vi "Get Exclusions.vi"(8 "error in (no error)":errorcluster, 11 "NI_AB_API_Build in":refnum<class "NI_AB_API_Build.lvclass">) -> (0 "error out":errorcluster, 1 "Disconnect inline subVIs":bool, 2 "Exclusions":T1, 3 "NI_AB_API_Build out":refnum<class "NI_AB_API_Build.lvclass">, 4 "Exclude dependent shared libraries":bool, 6 "Exclude dependent packed libraries":bool)   [LabVIEW 2020, in "NI_AB_API_Build.lvclass"]
uses:
  <vilib>/AppBuilder/AB_API/Build/NI_AB_API_Build.lvclass
  <vilib>/AppBuilder/AB_API/common/AB_API Primary Exclusions.ctl
  <vilib>/AppBuilder/AB_API/Build/NI_AB_API_Build.lvclass/NI_AB_API_Build.ctl
  <vilib>/AppBuilder/AB_Classes/Build/AB_Build.lvclass
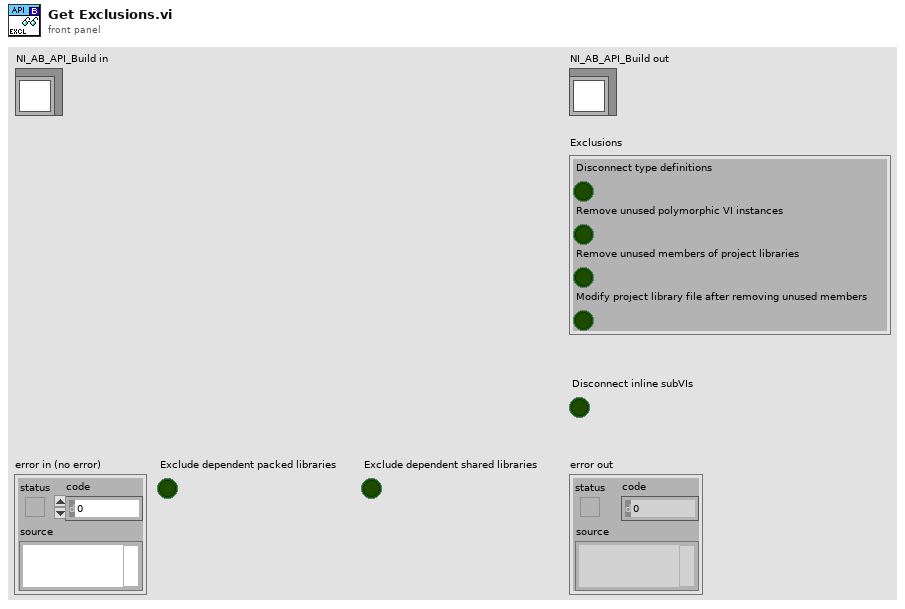
[diagram p1: front panel]
types:
  T1 = typedef "AB_API Primary Exclusions.ctl" = cluster{"Disconnect type definitions":bool, "Remove unused polymorphic VI instances":bool, "Remove unused members of project libraries":bool, "Modify project library file after removing unused members":bool}
  T2 = typedef "AB_Build.ctl" = cluster{"buildSpecName":string, "buildSpecDescription":string, "destinations":refnum<class "AB_Destination.lvclass">[], "exclusionOption":T3, "defaultLanguage":string, "supportedLanguages":string[], "excludedDirectories":path[], "buildContext":refnum<vi>, "buildObject":T4, "preview":bool, "programatic":bool, "progressBarEvents":T5, "userLog_Path":path, "preActionID":string, "preAction_Path":path, "postActionID":string, "postAction_Path":path, "eng_checkForBrokenVIs?":bool, "eng_verboseLinkerErrors?":bool, "localDest_Path":path, "targetDest_Path":path, "removeVIObject":u16, "cache":refnum<class "PreviewCache.lvclass">, "use cache":bool, "previewCache_ID":string, "buildCache_ID":string, "eng_TempLocalDest_Path":path, "eng_collectDependencies?":bool, "versionInfo":cluster{"buildVersion":cluster{"major":u16, "minor":u16, "patch":u16, "build":u16}, "autoIncrement":bool}, "eng_enableVIChecksums":bool}
  T3 = typedef "AB_Exclusion_Option.ctl" = cluster{"typedefs":bool, "polymorphicVIs":bool, "unusedLibraryItems":bool, "modifyLibraryFile":bool, "edit-timeDependencies":bool, "inlineVIs":bool, "dependent PPLs":bool, "dependent DLLs":bool}
  T4 = typedef "ItemRef.ctl" = u64
  T5 = typedef "provcom_ProgressBar_Events.ctl" = cluster{"newJob":refnum<user-event>, "newItem":refnum<user-event>, "errorMsg":T6, "cancel":refnum<user-event>}
  T6 = typedef "mxLvBuildError.ctl" = refnum<user-event>
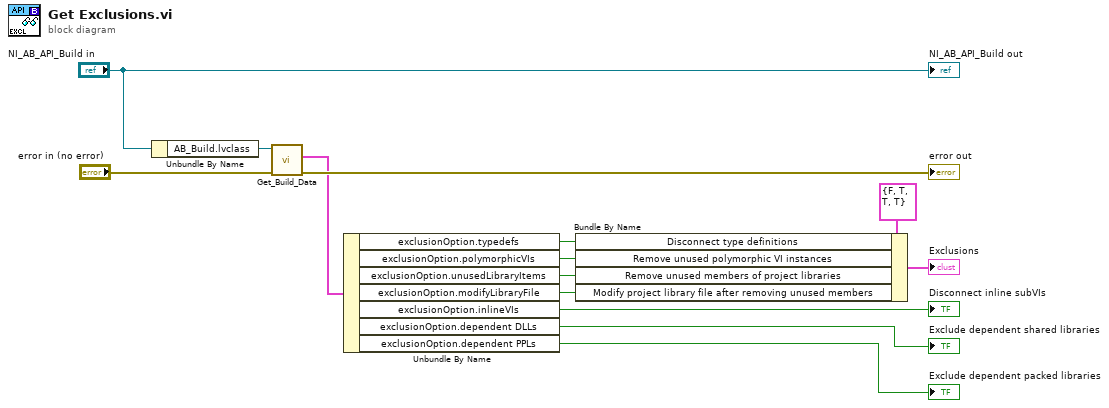
[diagram p0: block diagram]
diagram:
  n1 = Unbundle By Name("NI_AB_API_Build in") -> ("AB_Build.lvclass"=w13:refnum<class "AB_Build.lvclass">)
  n2 = call <vilib>:"Get_Build_Data.vi"("error in (no error)"="error in (no error)", "Class in"=w13) -> ("error out"=→"error out":errorcluster, "data"=w10:T2)  [unwired: 8 out]
  n3 = Unbundle By Name(w10) -> ("exclusionOption.typedefs"=w8:bool, "exclusionOption.polymorphicVIs"=w7:bool, "exclusionOption.unusedLibraryItems"=w6:bool, "exclusionOption.modifyLibraryFile"=w5:bool, "exclusionOption.inlineVIs"=→"Disconnect inline subVIs":bool, "exclusionOption.dependent DLLs"=→"Exclude dependent shared libraries":bool, "exclusionOption.dependent PPLs"=→"Exclude dependent packed libraries":bool)
  n4 = Bundle By Name(cluster=T1 {"Disconnect type definitions"=FALSE, "Remove unused polymorphic VI instances"=TRUE, "Remove unused members of project libraries"=TRUE, "Modify project library file after removing unused members"=TRUE} ("Exclusions"), "Disconnect type definitions"=w8, "Remove unused polymorphic VI instances"=w7, "Remove unused members of project libraries"=w6, "Modify project library file after removing unused members"=w5) -> (→"Exclusions":T1)
  "NI_AB_API_Build out" <- "NI_AB_API_Build in"
